vi "CreateExperimentRunTimingNode.vi"(8 "Error In":errorcluster, 10 "Experiment Run Timing":T1, 11 "DOM Document In":refnum<k20>) -> (0 "Error out":errorcluster, 2 "Experiment Run Timing Node":refnum<k20>, 3 "DOM Document Out":refnum<k20>)   [LabVIEW 2012]
uses:
  ExperimentRunTiming.ctl
  <resource>/objmgr/DOMUserDefRef.rc
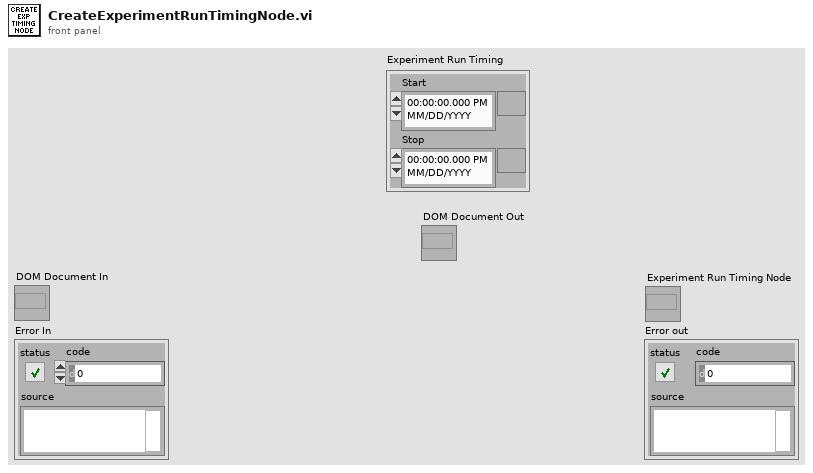
[diagram p1: front panel]
types:
  T1 = typedef "ExperimentRunTiming.ctl" = cluster{"Start":timestamp, "Stop":timestamp}
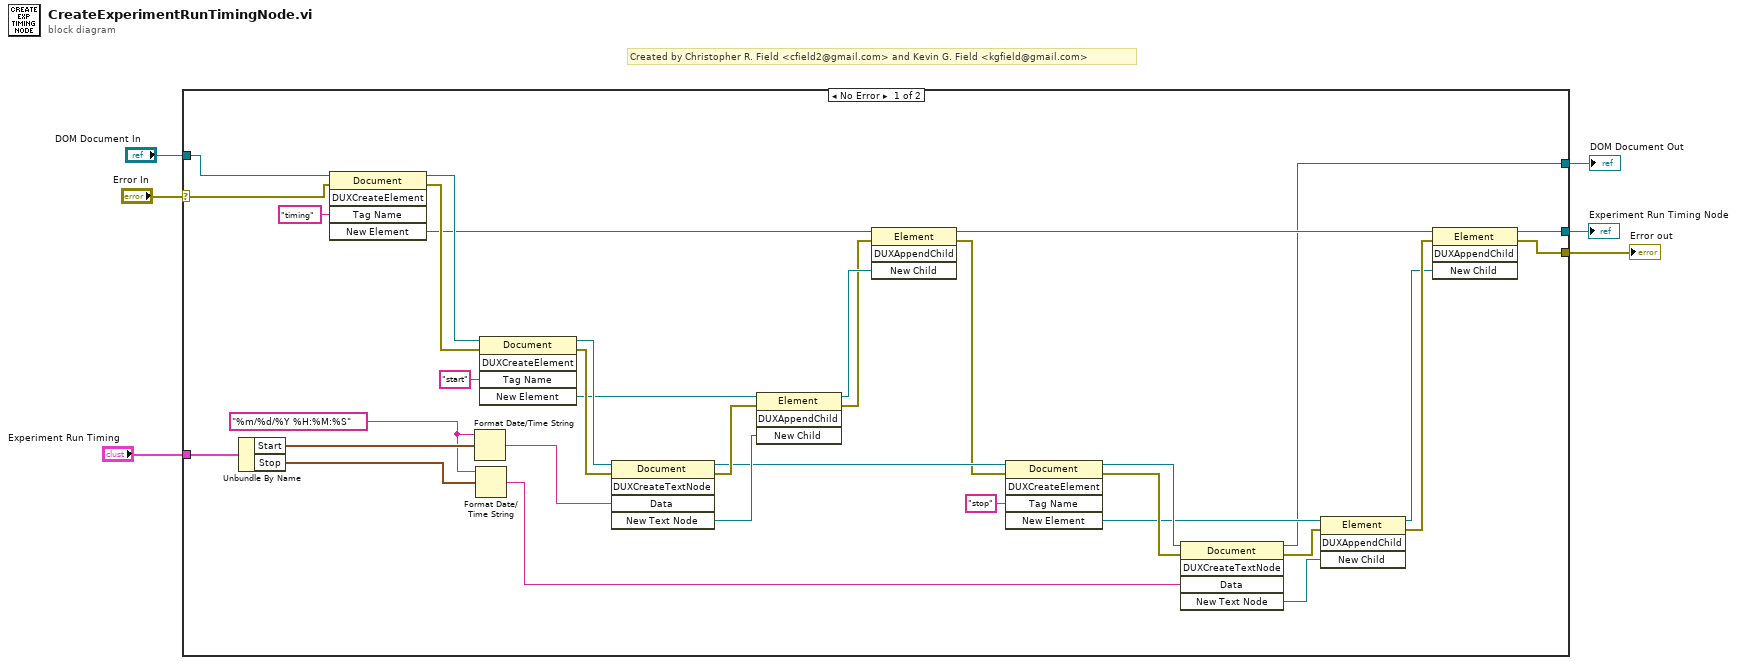
[diagram p0: block diagram]
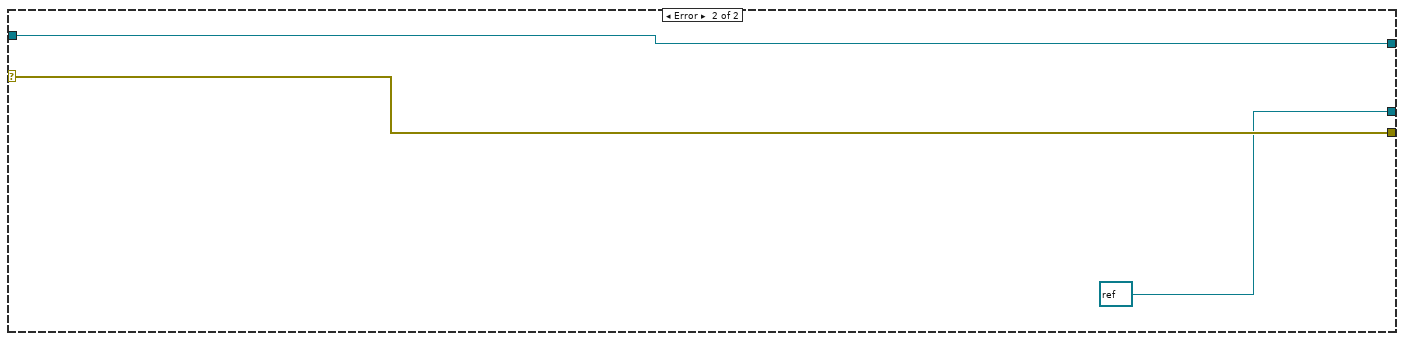
[diagram p2: hidden frame]
diagram:
  # "Created by Christopher R. Field <cfield2@gmail.com> and Kevin G. Field <kgfield@gmail.com>"
  n1 = case shown="No Error" "Error In" {
    selector: "Error In" -> [w37 w42]
    tunnel: "DOM Document In" -> [w40 w43]
    tunnel: [w9 refnum<k20> refnum ("Operator Node 2")] -> w5
    tunnel: [w7 w42] -> w4
    tunnel: [w8 w43] -> w2
    tunnel: "Experiment Run Timing" -> [w36 _]
    frame No Error {
      w27 = "%m/%d/%Y %H:%M:%S" ("time format string (%c)")
      n2 = Unbundle By Name(w36) -> ("Start"=w28:timestamp, "Stop"=w26:timestamp)
      n3 = invoke class="Document" method="DUXCreateElement"(reference=w40, error in=w37, "Tag Name"="timing") -> (reference out=w35:refnum<k20>, error out=w33:errorcluster, "New Element"=w23:refnum<k20>)  [unwired: 2 in, 2 out]
      n4 = Format Date/Time String(time format string (%c)=w27, seconds (now)=w28) -> (date/time string=w25:string)  [unwired: 1 in]
      n5 = Format Date/Time String(time format string (%c)=w27, seconds (now)=w26) -> (date/time string=w13:string)  [unwired: 1 in]
      n6 = invoke class="Document" method="DUXCreateElement"(reference=w35, error in=w33, "Tag Name"="start") -> (reference out=w32:refnum<k20>, error out=w31:errorcluster, "New Element"=w30:refnum<k20>)  [unwired: 2 in, 2 out]
      n7 = invoke class="Document" method="DUXCreateTextNode"(reference=w32, error in=w31, "Data"=w25) -> (reference out=w21:refnum<k20>, error out=w29:errorcluster, "New Text Node"=w38:refnum<k20>)  [unwired: 2 in, 2 out]
      n8 = invoke class="Element" method="DUXAppendChild"(reference=w30, error in=w29, "New Child"=w38) -> (reference out=w24:refnum<k20>, error out=w22:errorcluster)  [unwired: 1 in, 2 out]
      n9 = invoke class="Element" method="DUXAppendChild"(reference=w23, error in=w22, "New Child"=w24) -> (reference out=w10:refnum<k20>, error out=w20:errorcluster)  [unwired: 1 in, 2 out]
      n10 = invoke class="Document" method="DUXCreateElement"(reference=w21, error in=w20, "Tag Name"="stop") -> (reference out=w18:refnum<k20>, error out=w17:errorcluster, "New Element"=w16:refnum<k20>)  [unwired: 2 in, 2 out]
      n11 = invoke class="Document" method="DUXCreateTextNode"(reference=w18, error in=w17, "Data"=w13) -> (reference out=w8:refnum<k20>, error out=w15:errorcluster, "New Text Node"=w14:refnum<k20>)  [unwired: 2 in, 2 out]
      n12 = invoke class="Element" method="DUXAppendChild"(reference=w16, error in=w15, "New Child"=w14) -> (reference out=w11:refnum<k20>, error out=w12:errorcluster)  [unwired: 1 in, 2 out]
      n13 = invoke class="Element" method="DUXAppendChild"(reference=w10, error in=w12, "New Child"=w11) -> (reference out=w9:refnum<k20>, error out=w7:errorcluster)  [unwired: 1 in, 2 out]
    }
    frame Error {
    }
  }
  "Experiment Run Timing Node" <- w5
  "Error out" <- w4
  "DOM Document Out" <- w2
